vi "ConvertI16-U16Tiff_AllInPath.vi"() -> ()   [LabVIEW 2011]
panel:
  out "All Files":path[](array[path])
  out "Numeric":i32
  in  "pattern":string="*.tif"
  in  "Path":path
  # "connverts all files in directory to U16, sub vi can be used for conversion (bigtill, text..)"
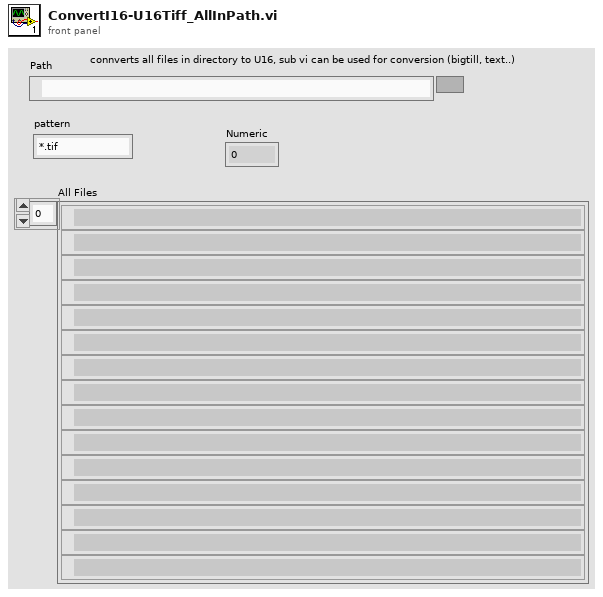
[diagram p1: front panel]
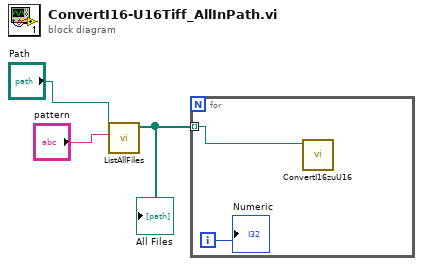
[diagram p0: block diagram]
diagram:
  n1 = call "ListAllFiles.vi"("pattern"="pattern", "vi path"="Path") -> ("All Files"=w1:path[])  [unwired: 8 in, 1 out]
  "All Files" <- w1
  n2 = for {
    tunnel: w1 -> [w5] mode=indexing
    i -> [w4]
    n3 = call "ConvertI16zuU16.vi"("file path"=w5) -> ()  [unwired: 7 in]
    "Numeric" <- w4
  }
